vi "Read notifierRef.vi"(8 "error in (no error)":errorcluster, 11 "NotifierStopMechanism in":refnum<class "BoolNotifierStopMechanism.lvclass">) -> (0 "error out":errorcluster, 2 "notifierRef":refnum<notifier>, 3 "NotifierStopMechanism out":refnum<class "BoolNotifierStopMechanism.lvclass">)   [LabVIEW 2023, in "TLC_Daemon.lvlib" / "BoolNotifierStopMechanism.lvclass"]
doc: "_____________________________________\nTLC Daemon 1.0.0.2\nCopyright (c) 2026 Andrea Cadei"
uses:
  BoolNotifierStopMech/BoolNotifierStopMechanism.lvclass
  BoolNotifierStopMech/BoolNotifierStopMechanism.lvclass/BoolNotifierStopMechanism.ctl
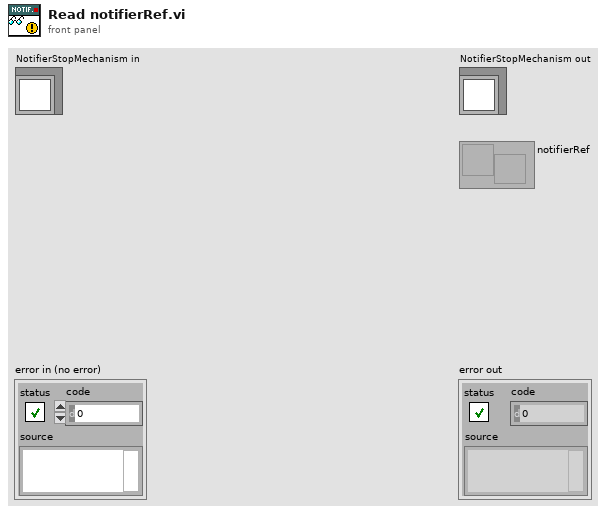
[diagram p1: front panel]
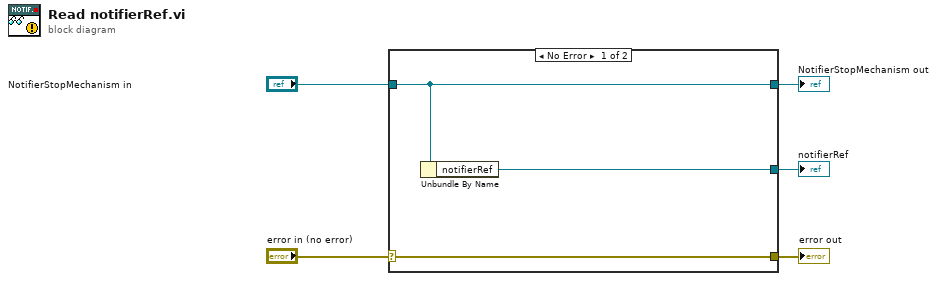
[diagram p0: block diagram]
diagram:
  n1 = case shown="No Error" "error in (no error)" {
    selector: "error in (no error)" -> [w8 w9]
    tunnel: [w8 w9] -> w4
    tunnel: [w7 w10] -> w2
    tunnel: "NotifierStopMechanism in" -> [w7 w10]
    tunnel: [w6 _] -> w1
    frame No Error {
      n2 = Unbundle By Name(w7) -> ("notifierRef"=w6:refnum<notifier>)
    }
    frame Error {
    }
  }
  "error out" <- w4
  "NotifierStopMechanism out" <- w2
  "notifierRef" <- w1
